vi "HMI.vi"(8 "error in (no error)":errorcluster caption="entrée d'erreur (pas d'erreur)", 11 "Class Popup Operator_Input (Default) en entrée":refnum<class "Class Popup Operator_Input (Default).lvclass">) -> (0 "error out":errorcluster caption="sortie d'erreur", 1 "Input":string="Attente \nvalidation", 2 "Operator_Selection":bool, 3 "Class Popup Operator_Input (Default) en sortie":refnum<class "Class Popup Operator_Input (Default).lvclass">)   [LabVIEW 2020, in "Library Instrument & Equipement.lvlib" / "Library Popup.lvlib" / "Class Popup Operator_Input (Default).lvclass"]
uses:
  Class Popup Operator_Input (Default).lvclass
  C:/Users/ngarcin/OneDrive - Altyor/Standard TB/Class/Popup/Class Popup (Main)/Class Popup (Main).lvclass
  Class Popup (Main)/Class Popup (Main).lvclass
  Class Popup Operator_Input (Default).lvclass/Class Popup Operator_Input (Default).ctl
panel:
  in  "Bouton NOK":bool
  in  "Input OP":string="Attente \nvalidation"
  in  "Bouton OK":bool
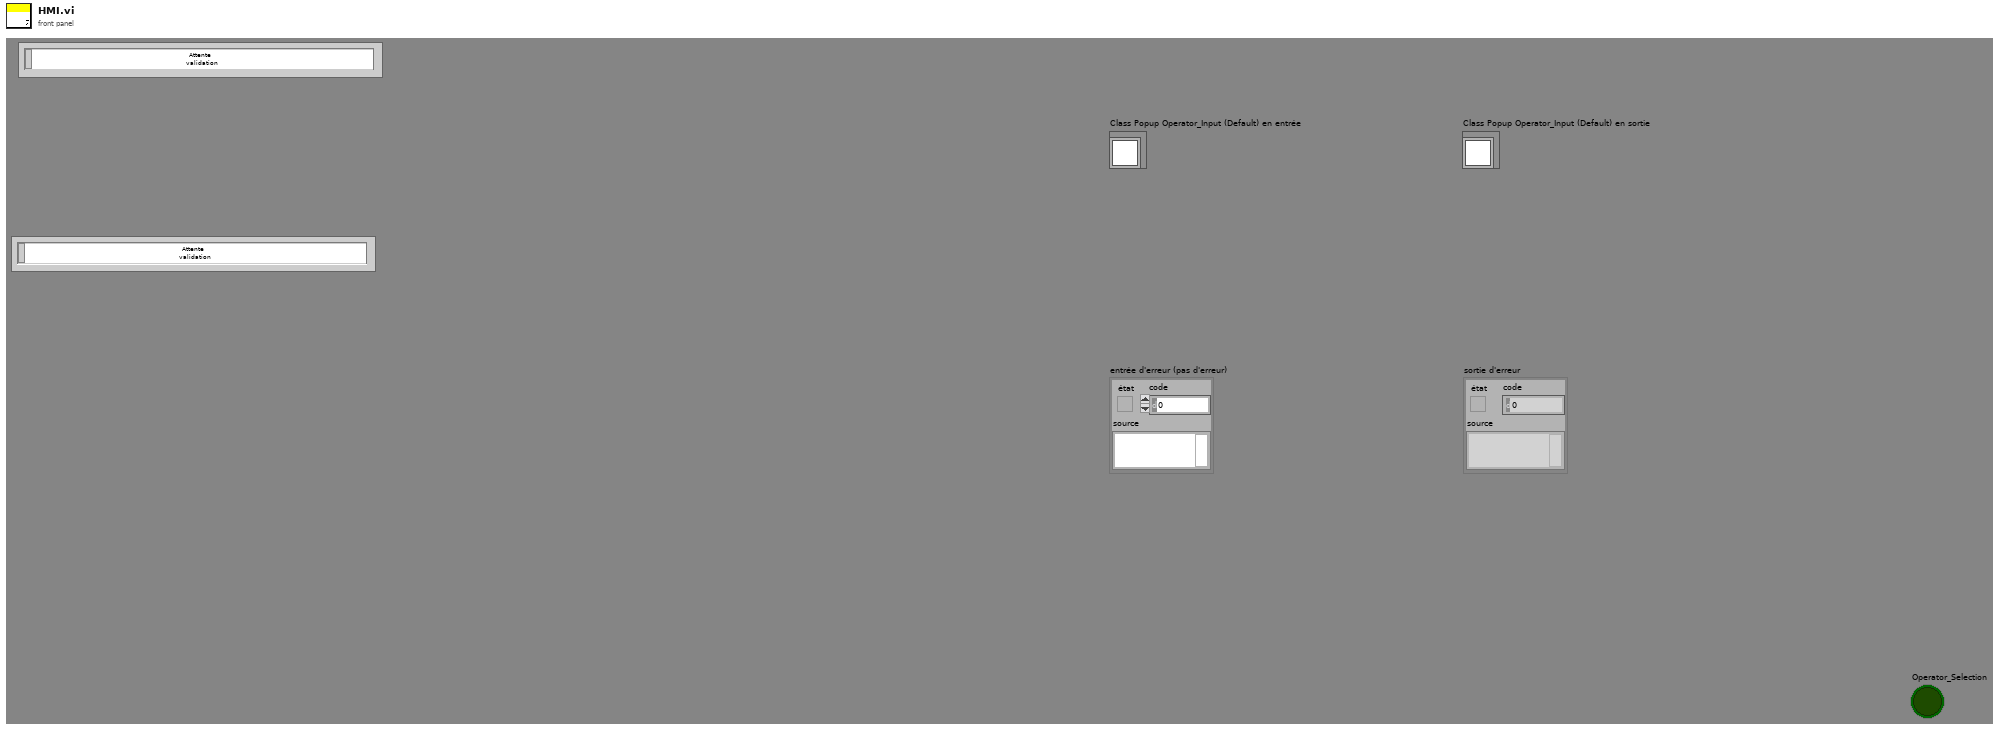
[diagram p1: front panel]
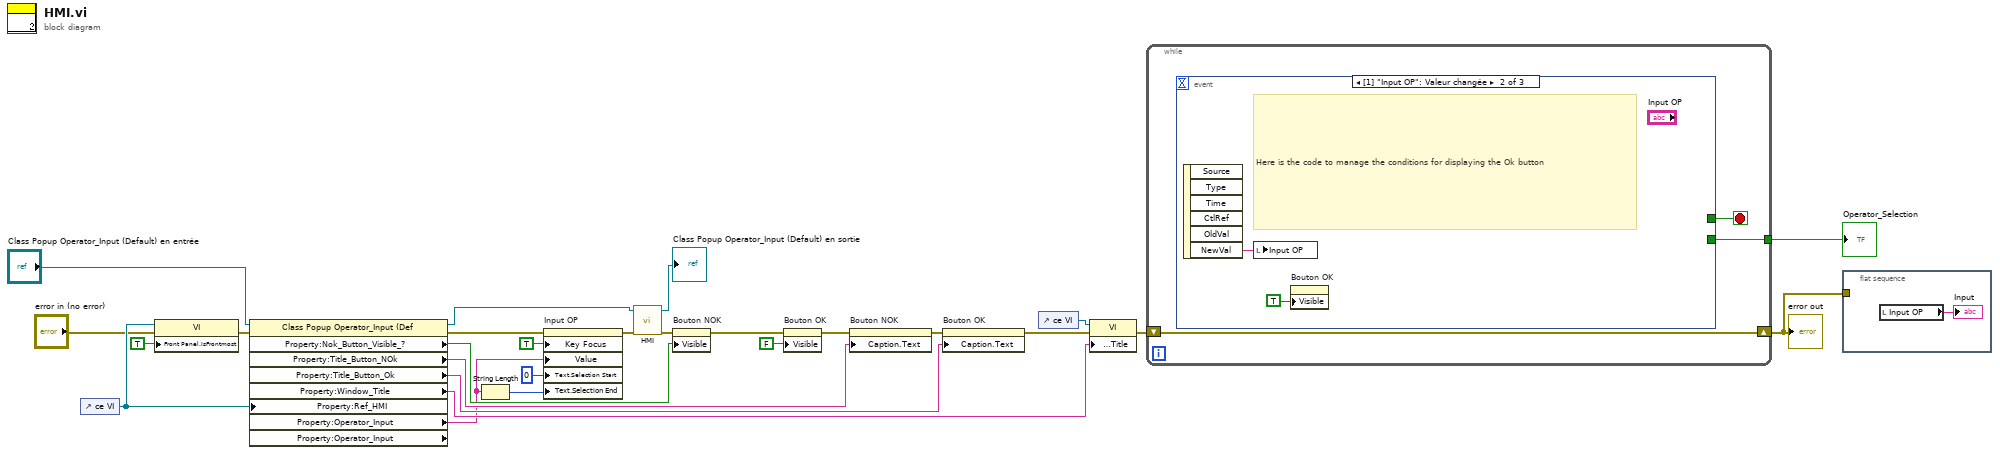
[diagram p0: block diagram]
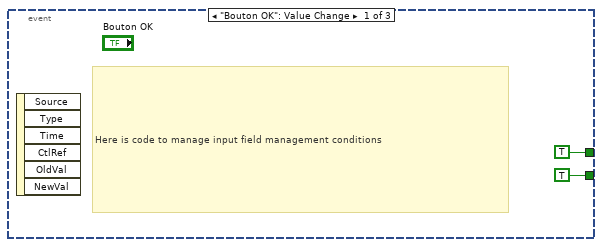
[diagram p2: hidden frame]
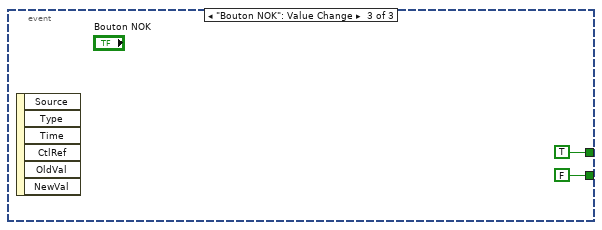
[diagram p3: hidden frame]
diagram:
  n1 = control-ref of="ce VI"() -> (w10:refnum<vi>)
  n2 = property class="VI"(reference=w10, error in="error in (no error)", "Front Panel.IsFrontmost"=TRUE ("Fenêtre face-avant:Au premier plan")) -> (error out=w8:errorcluster)  [unwired: 1 out]
  n3 = property class="Class Popup Operator_Input (Def" props=["Property:Nok_Button_Visible_?", "Property:Title_Button_NOk", "Property:Title_Button_Ok", "Property:Window_Title", "Property:Ref_HMI", "Property:Operator_Input", "Property:Operator_Input"](reference="Class Popup Operator_Input (Default) en entrée", error in=w8, "Property:Ref_HMI"=w10) -> (reference out=w21:refnum<class "Class Popup Operator_Input (Default).lvclass">, error out=w14:errorcluster, "Property:Nok_Button_Visible_?"=w27:bool, "Property:Title_Button_NOk"=w20:string, "Property:Title_Button_Ok"=w18:string, "Property:Window_Title"=w24:string, "Property:Operator_Input"=w5:string)  [unwired: 1 out]
  n4 = String Length(string=w5) -> (length=w7:i32)
  n5 = property on="Input OP" class="Ch"(error in=w14, "Key Focus"=TRUE ("Focus clavier"), "Value"=w5, "Text.Selection Start"=u32 0 ("Texte.Sélection:Début"), "Text.Selection End"=w7) -> (error out=w13:errorcluster)  [unwired: 1 in, 1 out]
  n6 = call-parent "HMI.vi"("error in (no error)"=w13, "Class Popup (Main) en entrée"=w21) -> ("error out"=w23:errorcluster, "Class Popup (Main) en sortie"=→"Class Popup Operator_Input (Default) en sortie":refnum<class "Class Popup Operator_Input (Default).lvclass">)  [unwired: 6 in, 2 out]
  n7 = property on="Bouton NOK" class="Bool"(error in=w23, "Visible"=w27) -> (error out=w16:errorcluster)  [unwired: 1 in, 1 out]
  n8 = property on="Bouton OK" class="Bool"(error in=w16, "Visible"=FALSE ("Activer ?")) -> (error out=w15:errorcluster)  [unwired: 1 in, 1 out]
  n9 = property on="Bouton NOK" class="Bool"(error in=w15, "Caption.Text"=w20) -> (error out=w19:errorcluster)  [unwired: 1 in, 1 out]
  n10 = property on="Bouton OK" class="Bool"(error in=w19, "Caption.Text"=w18) -> (error out=w11:errorcluster)  [unwired: 1 in, 1 out]
  n11 = control-ref of="ce VI"() -> (w25:refnum<vi>)
  n12 = property class="VI"(reference=w25, error in=w11, "Front Panel.Title"=w24) -> (error out=w22:errorcluster)  [unwired: 1 out]
  n13 = while {
    tunnel: [w28] -> w26
    shift-right: [w29] -> w4
    shift-left: w22 -> [w29]
    stop <- w30 stop-if-true
    n14 = event shown="[1] \"Input OP\": Valeur changée" {
      selector: _ -> [_ _ _]
      dyn-events: _ -> [_ _ _]
      timeout: _ -> [_ _ _]
      tunnel: [TRUE ("Valeur (Signalisation)") _ TRUE ("Valeur (Signalisation)")] -> w30
      tunnel: [TRUE ("Operator_Selection") _ FALSE ("Operator_Selection")] -> w28
      event "Bouton OK": Value Change {
        # "Here is code to manage input field management conditions"
        n15 = event-data() -> ()  [unwired: 1 in, 6 out]
      }
      event "Input OP": Value Change {
        # "Here is the code to manage the conditions for displaying the Ok button"
        n16 = event-data() -> ("NewVal"=w34:string)  [unwired: 1 in, 5 out]
        n17 = local write "Input OP"(w34) -> ()
        n18 = property on="Bouton OK" class="Bool"("Visible"=TRUE) -> ()  [unwired: 2 in, 2 out]
      }
      event "Bouton NOK": Value Change {
        n19 = event-data() -> ()  [unwired: 1 in, 6 out]
      }
    }
  }
  "error out" <- w4
  "Operator_Selection" <- w26
  n20 = flat-sequence {
    tunnel: w4 -> [_]
    frame #0 {
      n21 = local read "Input OP"() -> (→"Input":string)
    }
  }
